vi "Delete_Alone_101_from_Subtracks-2.vi"(4 "error IN":errorcluster, 5 "[IN] # of Correc\nted Longest Track":i32, 6 "[IN] # of Prob\nlem Point Inside":i32, 7 "[IN] Still connected\ntracks in group":T2) -> (0 "error OUT":errorcluster, 1 "[OUT] Special case: \nAlone 101 point":bool, 3 "[OUT] Clusters for Re\nconstructed Tracks":T1)   [LabVIEW 2013]
doc: "Subprogram corrects mistake: alone 101 point which connects with ending of other subtrack (so this problem can't be resolved: there doesn't exist any competing elongation)"
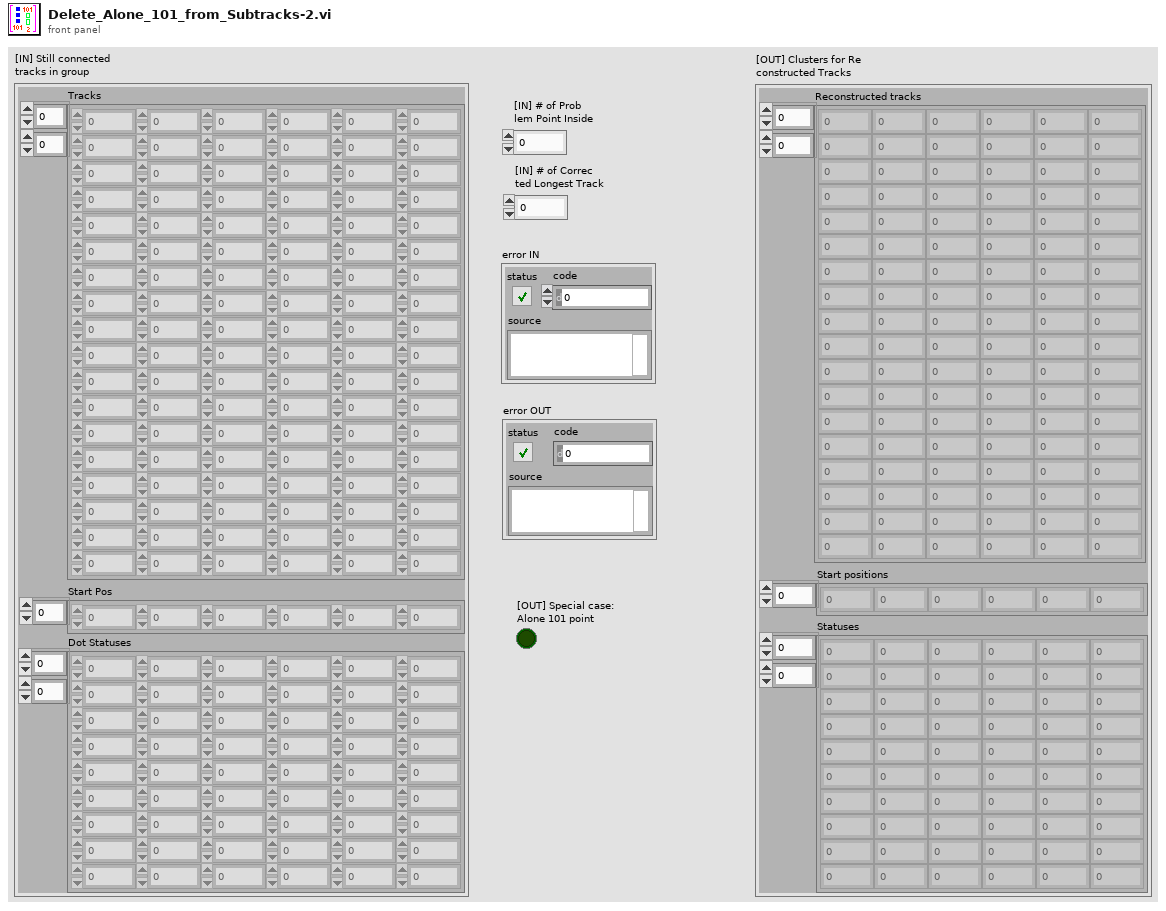
[diagram p1: front panel]
types:
  T1 = cluster{"Reconstructed tracks":dbl[][], "Start positions":i32[], "Statuses":i16[][]}
  T2 = cluster{"Tracks":dbl[][], "Start Pos":i32[], "Dot Statuses":i16[][]}
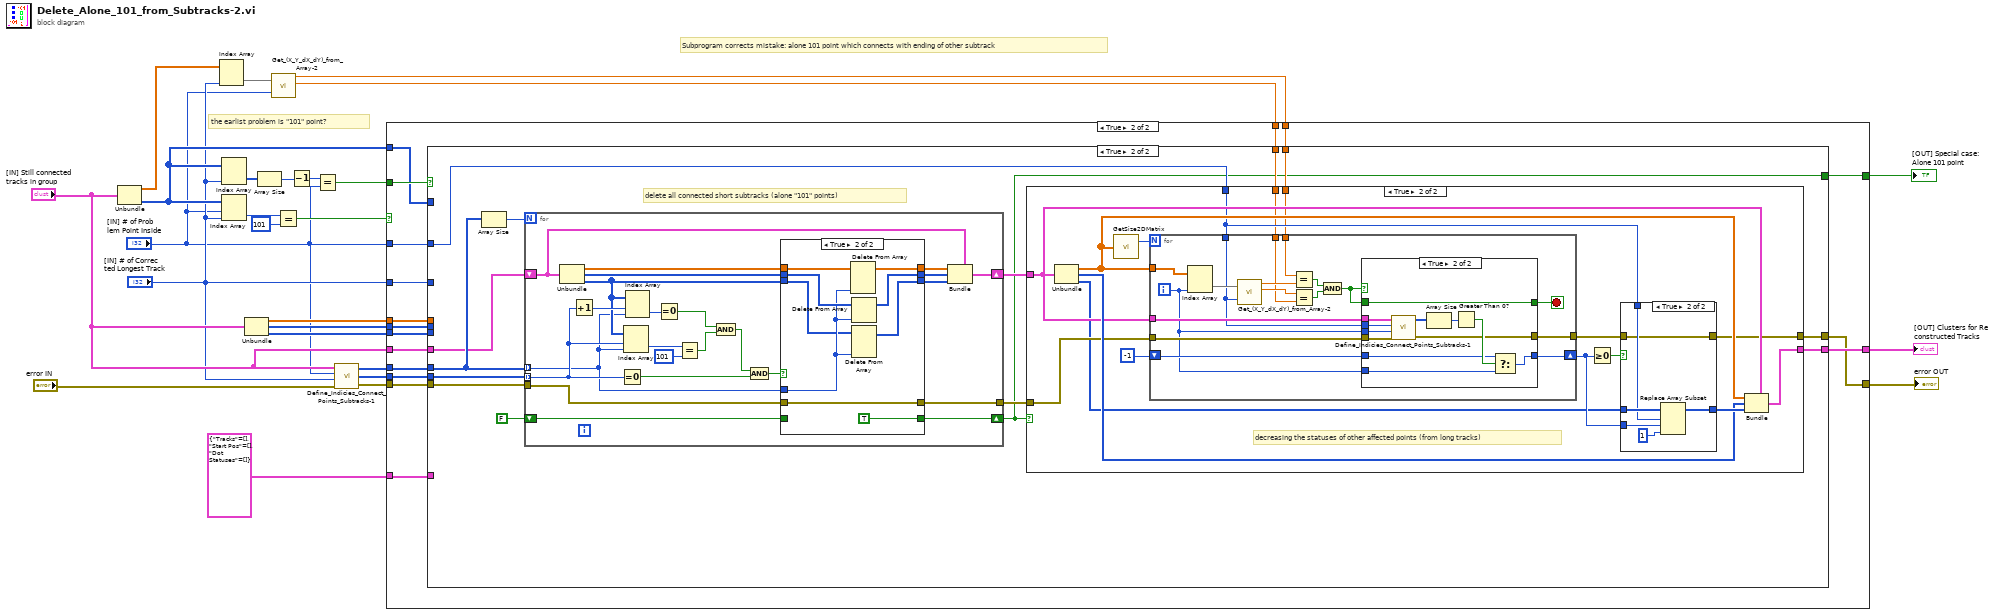
[diagram p0: block diagram]
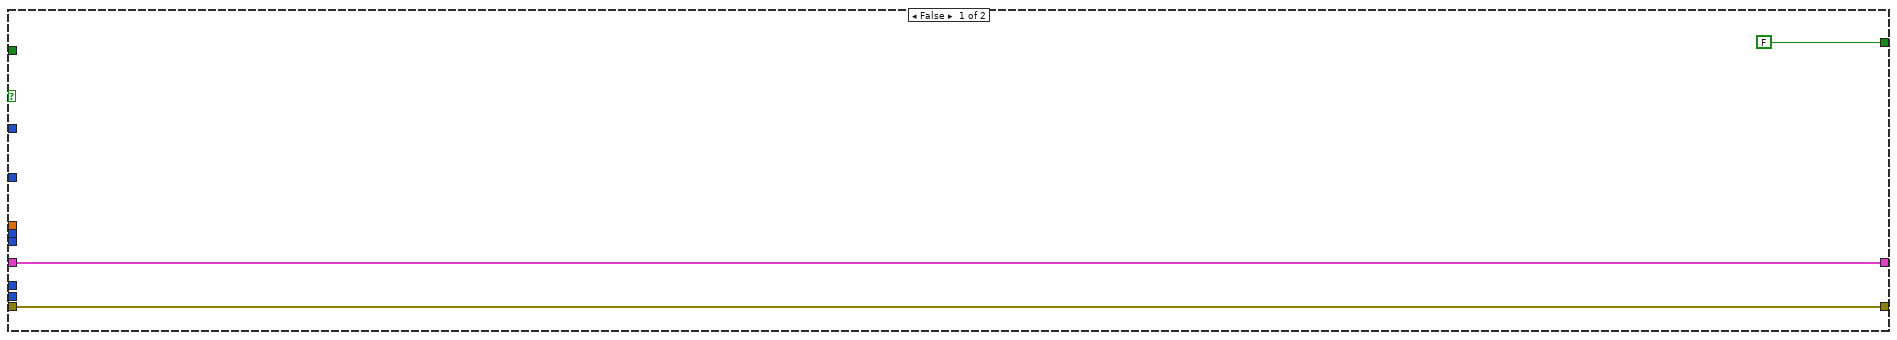
[diagram p2: hidden frame]
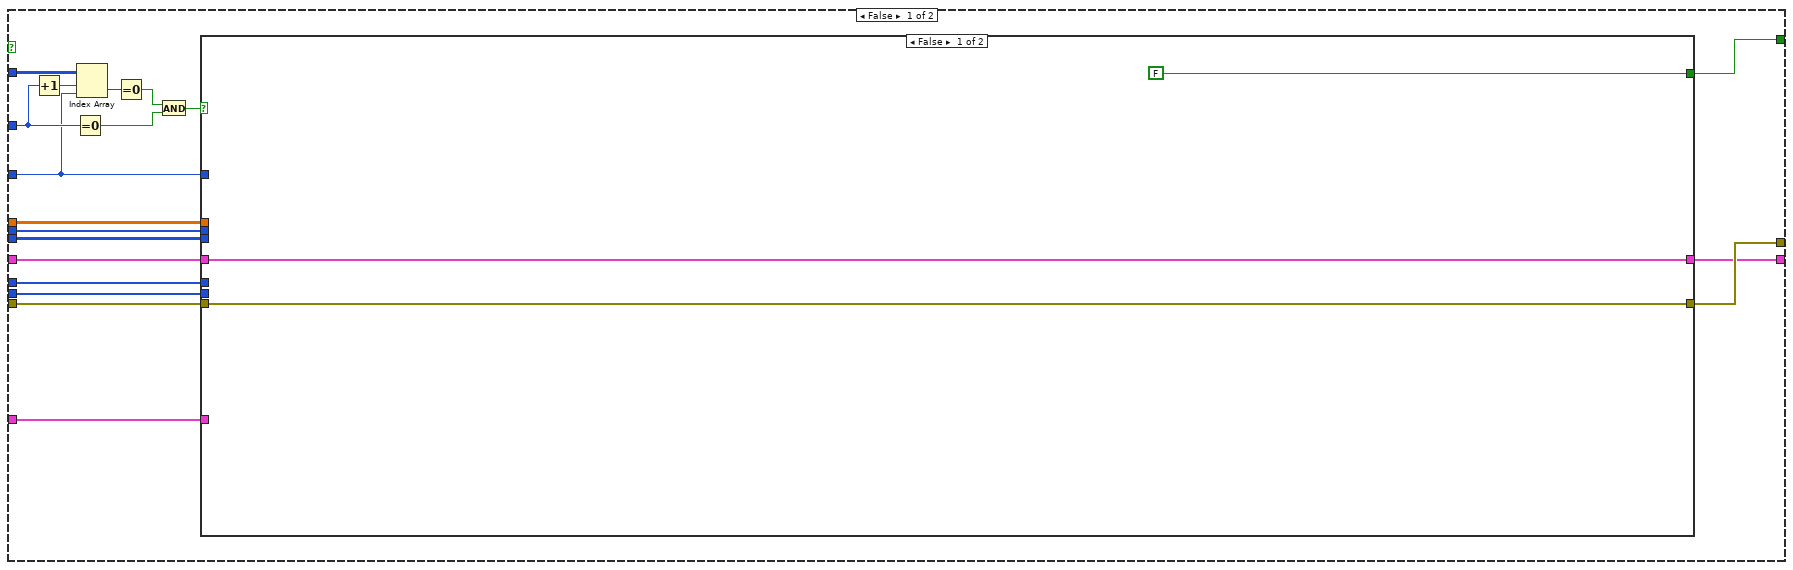
[diagram p3: hidden frame]
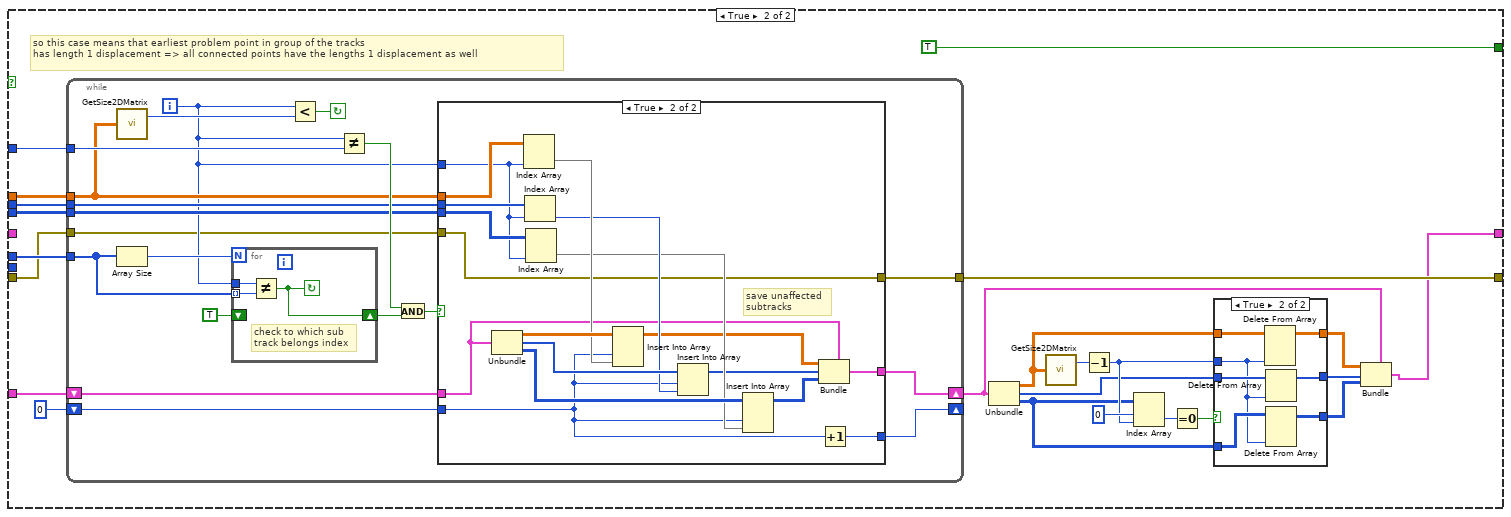
[diagram p4: hidden frame]
diagram:
  # "the earlist problem is \"101\" point?"
  # "Subprogram corrects mistake: alone 101 point which connects with ending of other subtrack"
  n1 = Unbundle("[IN] Still connected\ntracks in group") -> ("Tracks"=w9:dbl[][], "Dot Statuses"=w11:i16[][])  [unwired: 1 out]
  n2 = Index Array(array=w9, index (col)="[IN] # of Correc\nted Longest Track") -> (element=w7:dbl[])  [unwired: 1 in]
  n3 = Index Array(array=w11, index (col)="[IN] # of Correc\nted Longest Track") -> (element=w18:i16[])  [unwired: 1 in]
  n4 = Index Array(array=w11, index (row)="[IN] # of Prob\nlem Point Inside", index (col)="[IN] # of Correc\nted Longest Track") -> (element=w26:i16)
  n5 = Unbundle("[IN] Still connected\ntracks in group") -> ("Tracks"=w16:dbl[][], "Start Pos"=w15:i32[], "Dot Statuses"=w14:i16[][])
  n6 = Array Size(array=w18) -> (size(s)=w24:i32)
  n7 = call "Get_(X_Y_dX_dY)_from_Array-2.vi"("(X,Y,dX,dY)"=w7, "Index of Displacement"="[IN] # of Prob\nlem Point Inside") -> ("X"=w5:dbl, "Y"=w4:dbl)  [unwired: 2 out]
  n8 = Equal?(x=w26, y=i16 101) -> (x = y?=w13:bool)
  n9 = Decrement(x=w24) -> (x-1=w23:i32)
  n10 = Equal?(x=w23, y="[IN] # of Prob\nlem Point Inside") -> (x = y?=w12:bool)
  n11 = call "Define_Indicies_Connect_Points_Subtracks-1.vi"("error IN"="error IN", "[IN] Index of track with\n(problem displacement)"="[IN] # of Correc\nted Longest Track", "[IN] Index of problem\ndisplacement inside track"="[IN] # of Prob\nlem Point Inside", "[IN] Track group"="[IN] Still connected\ntracks in group") -> ("error OUT"=w19:errorcluster, "[OUT] Index of \nconnected dots\ninside the track"=w20:i32[], "[OUT] Index of connected\ntracks with problem dot"=w21:i32[])
  n12 = case shown="True" w13 {
    tunnel: w21 -> [_ w42]
    tunnel: w20 -> [_ w41]
    tunnel: w19 -> [w29 w36]
    tunnel: T2 {"Tracks"=[], "Start Pos"=[], "Dot Statuses"=[]} ("[IN] Still connected\ntracks in group") -> [_ w37]
    tunnel: w16 -> [_ w40]
    tunnel: "[IN] # of Correc\nted Longest Track" -> [_ w43]
    tunnel: w15 -> [_ w39]
    tunnel: w14 -> [_ w38]
    tunnel: w12 -> [_ w46]
    tunnel: w11 -> [_ w45]
    tunnel: "[IN] # of Prob\nlem Point Inside" -> [_ w44]
    tunnel: "[IN] Still connected\ntracks in group" -> [w27 w35]
    tunnel: w5 -> [_ w34]
    tunnel: w4 -> [_ w33]
    tunnel: [w29 w31] -> w2
    tunnel: [FALSE w30] -> w3
    tunnel: [w27 w32] -> w1
    frame False {
    }
    frame True {
      n13 = case shown="True" w46 {
        tunnel: w45 -> [w65 _]
        tunnel: w44 -> [w64 w150]
        tunnel: w43 -> [w55 _]
        tunnel: w42 -> [w58 w156]
        tunnel: w41 -> [w57 w155]
        tunnel: w40 -> [w56 _]
        tunnel: w39 -> [w54 _]
        tunnel: w38 -> [w53 _]
        tunnel: w37 -> [w52 _]
        tunnel: w36 -> [w50 w154]
        tunnel: w35 -> [w51 w153]
        tunnel: w34 -> [_ w149]
        tunnel: w33 -> [_ w148]
        tunnel: [w47 w147] -> w32
        tunnel: [w48 w146] -> w31
        tunnel: [w49 w145] -> w30
        frame False {
          n14 = Increment(x=w64) -> (x+1=w63:i32)
          n15 = Equal To 0?(x=w64) -> (x = 0?=w60:bool)
          n16 = Index Array(array=w65, index (row)=w63, index (col)=w55) -> (element=w62:i16)
          n17 = Equal To 0?(x=w62) -> (x = 0?=w61:bool)
          n18 = And(x=w61, y=w60) -> (x .and. y?=w59:bool)
          n19 = case shown="False" w59 {
            tunnel: w58 -> [_ w90]
            tunnel: w57 -> [_ _]
            tunnel: w56 -> [_ w91]
            tunnel: w55 -> [_ w89]
            tunnel: w54 -> [_ w88]
            tunnel: w53 -> [_ w87]
            tunnel: w52 -> [_ w86]
            tunnel: w51 -> [w68 _]
            tunnel: [w68 w69] -> w47
            tunnel: w50 -> [w67 w83]
            tunnel: [FALSE TRUE] -> w49
            tunnel: [w67 w72] -> w48
            frame False {
            }
            frame True {
              # "so this case means that earliest problem point in group of the tracks \nhas length 1 displacement => all connected points have the lengths 1 displacement as well"
              n20 = while {
                tunnel: w91 -> [w111]
                tunnel: w90 -> [w118]
                tunnel: w89 -> [w115]
                tunnel: w88 -> [w110]
                tunnel: w87 -> [w109]
                shift-right: [w105] -> w74
                shift-left: w86 -> [w108]
                shift-right: [w104] -> _
                shift-left: 0 -> [w107]
                tunnel: w83 -> [w103]
                tunnel: [w102] -> w72
                i -> [w106]
                stop <- w120 continue-if-true
                n21 = call "GetSize2DMatrix.vi"("Array IN (2D)"=w111) -> ("# Cols"=w116:i32)  [unwired: 1 out]
                n22 = Array Size(array=w118) -> (size(s)=w119:i32)
                n23 = for {
                  N: w119 -> [_]
                  tunnel: w118 -> [w143] mode=indexing
                  tunnel: w106 -> [w144]
                  shift-right: [w142] -> w113
                  shift-left: TRUE -> [_]
                  stop <- w142 continue-if-true
                  # "check to which sub\ntrack belongs index"
                  n24 = Not Equal?(x=w144, y=w143) -> (x != y?=w142:bool)
                }
                n25 = Less?(x=w106, y=w116) -> (x < y?=w120:bool)
                n26 = Not Equal?(x=w106, y=w115) -> (x != y?=w114:bool)
                n27 = And(x=w114, y=w113) -> (x .and. y?=w112:bool)
                n28 = case shown="True" w112 {
                  tunnel: w111 -> [_ w140]
                  tunnel: w110 -> [_ w138]
                  tunnel: w109 -> [_ w137]
                  tunnel: w108 -> [w123 w131]
                  tunnel: w107 -> [w122 w127]
                  tunnel: w106 -> [_ w136]
                  tunnel: [w122 w126] -> w104
                  tunnel: [w123 w125] -> w105
                  tunnel: w103 -> [w121 w124]
                  tunnel: [w121 w124] -> w102
                  frame False {
                  }
                  frame True {
                    # "save unaffected \nsubtracks"
                    n29 = Unbundle(w131) -> ("Tracks"=w141:dbl[][], "Start Pos"=w135:i32[], "Dot Statuses"=w133:i16[][])
                    n30 = Index Array(array=w140, index (col)=w136) -> (element=w139:dbl[])  [unwired: 1 in]
                    n31 = Index Array(array=w138, index=w136) -> (element=w134:i32)
                    n32 = Index Array(array=w137, index (col)=w136) -> (element=w132:i16[])  [unwired: 1 in]
                    n33 = Insert Into Array(array=w141, index (col)=w127, new element=w139) -> (w130:dbl[][])  [unwired: 1 in]
                    n34 = Insert Into Array(array=w135, index=w127, new element=w134) -> (w129:i32[])
                    n35 = Insert Into Array(array=w133, index (col)=w127, new element=w132) -> (w128:i16[][])  [unwired: 1 in]
                    n36 = Bundle(cluster=w131, "Tracks"=w130, "Start Pos"=w129, "Dot Statuses"=w128) -> (w125:T2)
                    n37 = Increment(x=w127) -> (x+1=w126:i32)
                  }
                }
              }
              n38 = Unbundle(w74) -> ("Tracks"=w78:dbl[][], "Start Pos"=w76:i32[], "Dot Statuses"=w75:i16[][])
              n39 = call "GetSize2DMatrix.vi"("Array IN (2D)"=w78) -> ("# Cols"=w82:i32)  [unwired: 1 out]
              n40 = Decrement(x=w82) -> (x-1=w77:i32)
              n41 = Index Array(array=w75, index (row)=0 ("disabled index (row)"), index (col)=w77) -> (element=w80:i16)
              n42 = Equal To 0?(x=w80) -> (x = 0?=w79:bool)
              n43 = case shown="True" w79 {
                tunnel: w78 -> [w94 w101]
                tunnel: w77 -> [_ w98]
                tunnel: w76 -> [w93 w100]
                tunnel: w75 -> [w92 w99]
                tunnel: [w94 w97] -> w73
                tunnel: [w93 w96] -> w71
                tunnel: [w92 w95] -> w70
                frame False {
                }
                frame True {
                  n44 = Delete From Array(array=w101, index (col)=w98) -> (array with subset deleted=w97:dbl[][])  [unwired: 2 in, 1 out]
                  n45 = Delete From Array(array=w100, index=w98) -> (array with subset deleted=w96:i32[])  [unwired: 1 in, 1 out]
                  n46 = Delete From Array(array=w99, index (col)=w98) -> (array with subset deleted=w95:i16[][])  [unwired: 2 in, 1 out]
                }
              }
              n47 = Bundle(cluster=w74, "Tracks"=w73, "Start Pos"=w71, "Dot Statuses"=w70) -> (w69:T2)
            }
          }
        }
        frame True {
          # "delete all connected short subtracks (alone \"101\" points)"
          n48 = Array Size(array=w156) -> (size(s)=w158:i32)
          n49 = for {
            N: w158 -> [_]
            shift-right: [w220] -> w151
            shift-left: w153 -> [w222]
            tunnel: w156 -> [w225] mode=indexing
            tunnel: w155 -> [w235] mode=indexing
            tunnel: w154 -> [w226]
            shift-right: [w223] -> w145
            shift-left: FALSE -> [w224]
            tunnel: [w217] -> w152
            n50 = Unbundle(w222) -> ("Tracks"=w229:dbl[][], "Start Pos"=w228:i32[], "Dot Statuses"=w227:i16[][])
            n51 = Increment(x=w235) -> (x+1=w237:i32)
            n52 = Equal To 0?(x=w235) -> (x = 0?=w238:bool)
            n53 = Index Array(array=w227, index (row)=w235, index (col)=w225) -> (element=w234:i16)
            n54 = Index Array(array=w227, index (row)=w237, index (col)=w225) -> (element=w239:i16)
            n55 = Equal To 0?(x=w239) -> (x = 0?=w233:bool)
            n56 = Equal?(x=w234, y=i16 101) -> (x = y?=w232:bool)
            n57 = And(x=w233, y=w232) -> (x .and. y?=w231:bool)
            n58 = And(x=w231, y=w238) -> (x .and. y?=w230:bool)
            n59 = case shown="True" w230 {
              tunnel: w229 -> [w244 w253]
              tunnel: w228 -> [w243 w252]
              tunnel: w227 -> [w242 w245]
              tunnel: w226 -> [w240 w247]
              tunnel: w225 -> [_ w251]
              tunnel: [w244 w250] -> w221
              tunnel: w224 -> [w241 _]
              tunnel: [w243 w249] -> w219
              tunnel: [w242 w246] -> w218
              tunnel: [w241 TRUE] -> w223
              tunnel: [w240 w247] -> w217
              frame False {
              }
              frame True {
                n60 = Delete From Array(array=w253, index (col)=w251) -> (array with subset deleted=w250:dbl[][])  [unwired: 2 in, 1 out]
                n61 = Delete From Array(array=w252, index=w251) -> (array with subset deleted=w249:i32[])  [unwired: 1 in, 1 out]
                n62 = Delete From Array(array=w245, index (col)=w251) -> (array with subset deleted=w246:i16[][])  [unwired: 2 in, 1 out]
              }
            }
            n63 = Bundle(cluster=w222, "Tracks"=w221, "Start Pos"=w219, "Dot Statuses"=w218) -> (w220:T2)
          }
          n64 = case shown="True" w145 {
            tunnel: w152 -> [w160 w168]
            tunnel: w151 -> [w159 w167]
            tunnel: w150 -> [_ w165]
            tunnel: w149 -> [_ w164]
            tunnel: w148 -> [_ w163]
            tunnel: [w159 w162] -> w147
            tunnel: [w160 w161] -> w146
            frame False {
            }
            frame True {
              # "decreasing the statuses of other affected points (from long tracks)"
              n65 = Unbundle(w167) -> ("Tracks"=w170:dbl[][], "Start Pos"=w169:i32[], "Dot Statuses"=w166:i16[][])
              n66 = call "GetSize2DMatrix.vi"("Array IN (2D)"=w170) -> ("# Cols"=w176:i32)  [unwired: 1 out]
              n67 = for {
                N: w176 -> [_]
                tunnel: w170 -> [w201]
                tunnel: w165 -> [w191]
                tunnel: w164 -> [w199]
                tunnel: w163 -> [w196]
                shift-right: [w186] -> w173
                shift-left: -1 -> [w188]
                tunnel: w167 -> [w193]
                tunnel: w168 -> [w192]
                tunnel: [w185] -> w171
                i -> [w187]
                stop <- w189 stop-if-true
                n68 = Index Array(array=w201, index (col)=w187) -> (element=w200:dbl[])  [unwired: 1 in]
                n69 = call "Get_(X_Y_dX_dY)_from_Array-2.vi"("(X,Y,dX,dY)"=w200, "Index of Displacement"=w191) -> ("X"=w198:dbl, "Y"=w197:dbl)  [unwired: 2 out]
                n70 = Equal?(x=w199, y=w198) -> (x = y?=w195:bool)
                n71 = Equal?(x=w197, y=w196) -> (x = y?=w194:bool)
                n72 = And(x=w195, y=w194) -> (x .and. y?=w190:bool)
                n73 = case shown="True" w190 {
                  tunnel: w193 -> [_ w216]
                  tunnel: w192 -> [w202 w215]
                  tunnel: w187 -> [_ w214]
                  tunnel: w191 -> [_ w213]
                  tunnel: w190 -> [w204 w212]
                  tunnel: [w204 w212] -> w189
                  tunnel: w188 -> [w203 w208]
                  tunnel: w187 -> [_ w207]
                  tunnel: [w203 w206] -> w186
                  tunnel: [w202 w205] -> w185
                  frame False {
                  }
                  frame True {
                    n74 = call "Define_Indicies_Connect_Points_Subtracks-1.vi"("error IN"=w215, "[IN] Index of track with\n(problem displacement)"=w214, "[IN] Index of problem\ndisplacement inside track"=w213, "[IN] Track group"=w216) -> ("error OUT"=w205:errorcluster, "[OUT] Index of connected\ntracks with problem dot"=w211:i32[])  [unwired: 1 out]
                    n75 = Array Size(array=w211) -> (size(s)=w210:i32)
                    n76 = Greater Than 0?(x=w210) -> (x > 0?=w209:bool)
                    n77 = Select(t=w208, s=w209, f=w207) -> (s? t:f=w206:i32)
                  }
                }
              }
              n78 = Greater Or Equal To 0?(x=w173) -> (x >= 0?=w174:bool)
              n79 = case shown="True" w174 {
                tunnel: w166 -> [w178 w184]
                tunnel: w173 -> [_ w183]
                tunnel: w165 -> [_ w182]
                tunnel: [w178 w180] -> w172
                tunnel: w171 -> [w177 w179]
                tunnel: [w177 w179] -> w161
                frame False {
                }
                frame True {
                  n80 = Replace Array Subset(array=w184, new element=i16 1 ("new element/subarray"), index (row)=w182, index (col)=w183) -> (w180:i16[][])
                }
              }
              n81 = Bundle(cluster=w167, "Tracks"=w170, "Start Pos"=w169, "Dot Statuses"=w172) -> (w162:T2)
            }
          }
        }
      }
    }
  }
  "[OUT] Clusters for Re\nconstructed Tracks" <- w1
  "error OUT" <- w2
  "[OUT] Special case: \nAlone 101 point" <- w3
